vi "Request Data.vi"(6 "Qualifier":string, 8 "error in":errorcluster, 9 "notifier":refnum<notifier>, 10 "Data to Send":string, 11 "DIG_IO in":refnum<class "DIG_IO.lvclass">) -> (0 "error out":errorcluster, 3 "DIG_IO out":refnum<class "DIG_IO.lvclass">)   [LabVIEW 2019, in "DIG_IO.lvlib" / "DIG_IO.lvclass"]
uses:
  Library/DIG_IO.lvclass
  C:/Users/Public/Documents/Development/builds/Instruments/Instruments.lvlibp/Library/Instruments.lvclass
  builds/Instruments/Instruments.lvlibp/Private/Accessors/Read Poll(ms).vi
  builds/Instruments/Instruments.lvlibp/Private/Polymorphic/Special/Event from String.vi
  builds/Instruments/Instruments.lvlibp/Accessors/Command with Logging.vi
  builds/Instruments/Instruments.lvlibp/Library/Instruments.lvclass
  builds/Instruments/Instruments.lvlibp
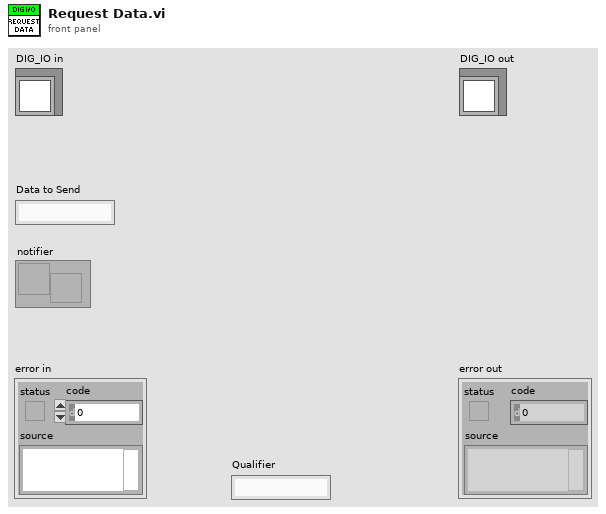
[diagram p1: front panel]
types:
  T1 = cluster{"Timestamp":timestamp, "Description":string, "Data":string}
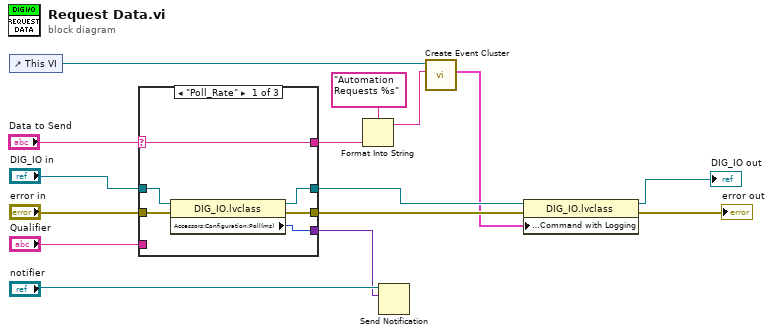
[diagram p0: block diagram]
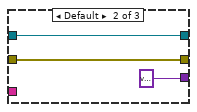
[diagram p2: hidden frame]
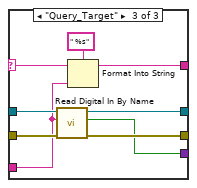
[diagram p3: hidden frame]
diagram:
  n1 = control-ref of="This VI"() -> (w3:refnum<vi>)
  n2 = case shown="\"Poll_Rate\"" "Data to Send" {
    selector: "Data to Send" -> [w21 _ w28]
    tunnel: "DIG_IO in" -> [w20 w24 w33]
    tunnel: [w19 w24 w32] -> w9
    tunnel: "error in" -> [w18 w23 w31]
    tunnel: [w17 w23 w30] -> w7
    tunnel: [w16 variant w29] -> w12
    tunnel: "Qualifier" -> [_ _ w26]
    tunnel: [w21 _ w25] -> w4
    frame "Poll_Rate" {
      n3 = property class="DIG_IO.lvclass"(reference=w20, error in=w18) -> (reference out=w19:refnum<class "DIG_IO.lvclass">, error out=w17:errorcluster, "Accessors:Configuration:Poll(ms)"=w16:u32)
    }
    frame Default {
    }
    frame "Query_Target" {
      n4 = call "Read Digital In By Name.vi"("error in"=w31, "Name"=w26, "DIG_IO in"=w33) -> ("error out"=w30:errorcluster, "State"=w29:bool, "DIG_IO out"=w32:refnum<class "DIG_IO.lvclass">)  [unwired: 6 in]
      n5 = Format Into String(format string=" %s", initial string=w28, w26) -> (resulting string=w25:string)  [unwired: 1 in, 1 out]
    }
  }
  n6 = Format Into String(format string="Automation Requests %s", w4) -> (resulting string=w2:string)  [unwired: 2 in, 1 out]
  n7 = Send Notification(notification=w12, notifier="notifier") -> ()  [unwired: 1 in, 2 out]
  n8 = call-poly "Create Event Cluster.vi"("Value"=w2, "VI Refnum"=w3) -> ("Event Data"=w1:T1)  [unwired: 9 in]
  n9 = property class="DIG_IO.lvclass"(reference=w9, error in=w7, "Accessors:Logging:Command with Logging"=w1) -> (reference out=→"DIG_IO out":refnum<class "DIG_IO.lvclass">, error out=→"error out":errorcluster)
